vi "Query Resource Access Information - NPin 1Rsrc.vi"(7 "sites":i32[](array[numeric]), 8 "error in (no error)":errorcluster, 9 "instrument type id":string, 10 "pin or relay names":string[](array[string]), 11 "pin map id":string) -> (0 "error out":errorcluster, 2 "resource access information":T1)   [LabVIEW 2020, in "MeasurementLink Pin Map.lvlib"]
doc: "Queries the pin map service for resouce access information for the specified <b>pin or relay names</b>, <b>instrument type</b>, and <b>sites</b>. This information can be used to map pins to the single hardware resource used to make measurements on the pins."
uses:
  MeasurementLink Pin Map.lvlib
  MeasurementLink Pin Map Client/RPC Messages/ni_measurementlink_pinmap_v1_ResourceAccessInformation.ctl
  MeasurementLink Pin Map Client/RPC Messages/ni_measurementlink_pinmap_v1_ChannelMapping.ctl
  MeasurementLink Pin Map Client/MeasurementLink Pin Map Client.lvlib
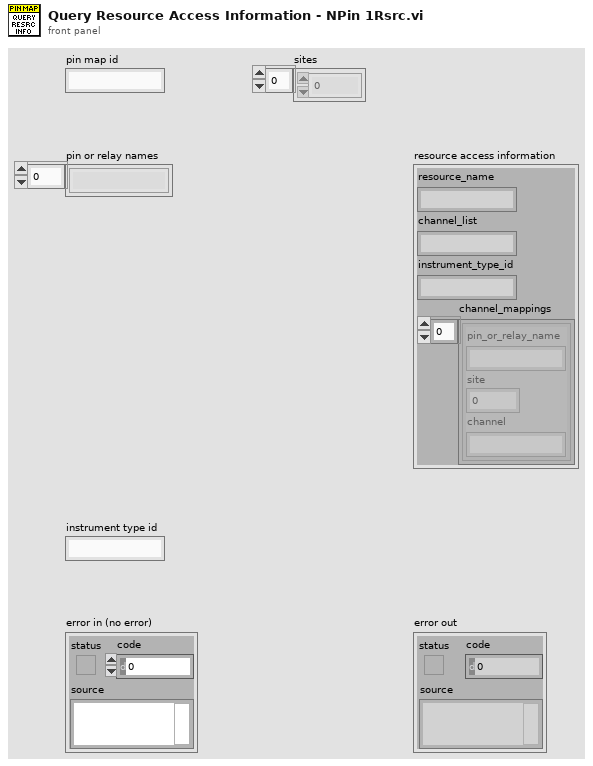
[diagram p1: front panel]
types:
  T1 = typedef "MeasurementLink Pin Map Client.lvlib/ni_measurementlink_pinmap_v1_ResourceAccessInformation.ctl" = cluster{"resource_name":string, "channel_list":string, "instrument_type_id":string, "channel_mappings":T2[]}
  T2 = typedef "MeasurementLink Pin Map Client.lvlib/ni_measurementlink_pinmap_v1_ChannelMapping.ctl" = cluster{"pin_or_relay_name":string, "site":i32, "channel":string}
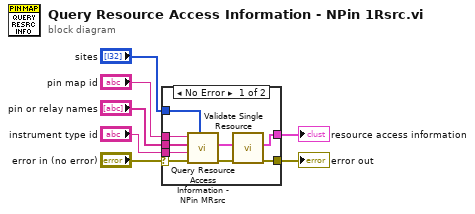
[diagram p0: block diagram]
diagram:
  n1 = case shown="No Error" "error in (no error)" {
    selector: "error in (no error)" -> [w16 w17]
    tunnel: "pin or relay names" -> [w14 _]
    tunnel: "instrument type id" -> [w15 _]
    tunnel: [w10 w17] -> w5
    tunnel: [w8 _] -> w3
    tunnel: "pin map id" -> [w13 _]
    tunnel: "sites" -> [w12 _]
    frame No Error {
      n2 = call "Query Resource Access Information - NPin MRsrc.vi"("sites"=w12, "error in (no error)"=w16, "instrument type id"=w15, "pin or relay names"=w14, "pin map id"=w13) -> ("error out"=w11:errorcluster, "resource access information"=w9:T1[])  [unwired: 5 in]
      n3 = call "Validate Single Resource.vi"("error in (no error)"=w11, "resources"=w9) -> ("error out"=w10:errorcluster, "resource"=w8:T1)  [unwired: 8 in]
    }
    frame Error {
    }
  }
  "error out" <- w5
  "resource access information" <- w3
